vi "Schreiben_verknuepfen.vi"(8 "error in (no error)":errorcluster caption="Fehler (Eingang, kein Fehler)", 10 "Order":string, 11 "Zahl":dbl) -> (0 "error out":errorcluster caption="Fehler (Ausgang)", 3 "Verknüpfter String":string)   [LabVIEW 2020, in "Linearisierung v2.lvlib" / "Gasteiler.lvlib" / "HovaCal.lvlib"]
uses:
  HovaCal.lvlib
panel:
  in  "Zieladresse":string="FF"
  in  "Quelladresse":string="00"
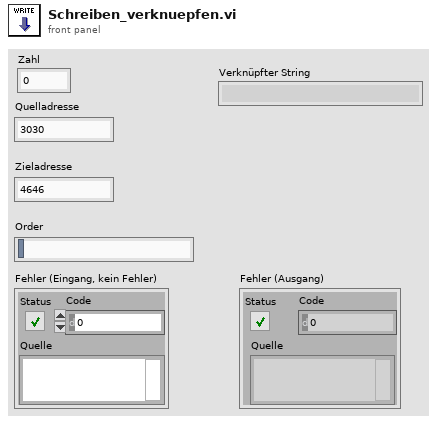
[diagram p1: front panel]
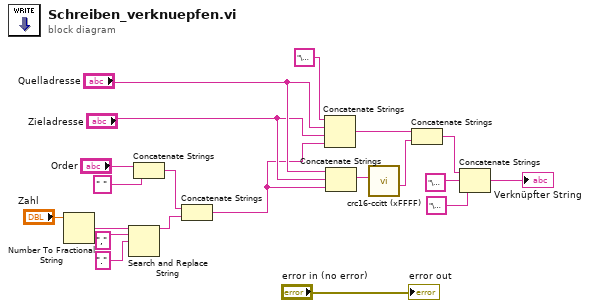
[diagram p0: block diagram]
diagram:
  n1 = Number To Fractional String(number="Zahl") -> (F-format string=w8:string)  [unwired: 3 in]
  n2 = Search and Replace String(input string=w8, search string="," ("Such-String"), replace string="." ("Ersetzungs-String (\"\")")) -> (result string=w5:string)  [unwired: 5 in, 3 out]
  n3 = Concatenate Strings("Order", " " ("String")) -> (w3:string)
  n4 = Concatenate Strings(w3, w5) -> (w4:string)
  n5 = Concatenate Strings("\u0002", "Quelladresse", "Zieladresse", w4) -> (w14:string)
  n6 = Concatenate Strings("Quelladresse", "Zieladresse", w4) -> (w12:string)
  n7 = call "crc16-ccitt (xFFFF).vi"("Message"=w12) -> ("Hex-Integer-String"=w11:string)  [unwired: 8 in, 2 out]
  n8 = Concatenate Strings(w14, w11) -> (w17:string)
  n9 = Concatenate Strings(w17, "\u0003", "\u0006" ("String")) -> (→"Verknüpfter String":string)
  "error out" <- "error in (no error)"
